vi "Read target.vi"(8 "error in (no error)":errorcluster, 11 "GuideTargetPosition in":refnum<class "GuideTargetPosition.lvclass">) -> (0 "error out":errorcluster, 2 "GWTargetPositionParameters.lvclass":refnum<class "GWTargetPositionParameters.lvclass">, 3 "GuideTargetPosition out":refnum<class "GuideTargetPosition.lvclass">)   [LabVIEW 2014, in "TCSDataDefinitions.lvlib" / "TCSGuiderStatus.lvlib" / "GuideTargetPosition.lvclass"]
uses:
  GuideTargetPosition.lvclass
  GWTargetPositionParameters/GWTargetPositionParameters.lvclass
  GuideTargetPosition.lvclass/GuideTargetPosition.ctl
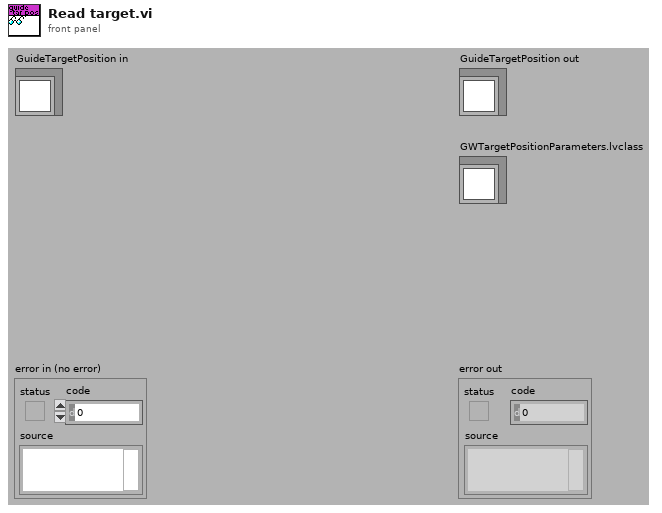
[diagram p1: front panel]
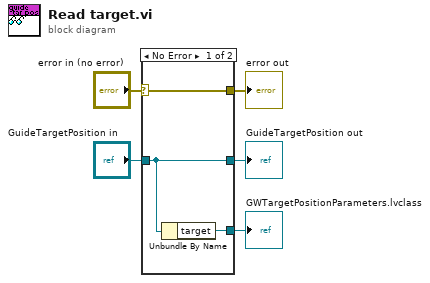
[diagram p0: block diagram]
diagram:
  n1 = case shown="No Error" "error in (no error)" {
    selector: "error in (no error)" -> [w8 w9]
    tunnel: [w8 w9] -> w4
    tunnel: [w7 w10] -> w2
    tunnel: "GuideTargetPosition in" -> [w7 w10]
    tunnel: [w6 _] -> w1
    frame No Error {
      n2 = Unbundle By Name(w7) -> ("target"=w6:refnum<class "GWTargetPositionParameters.lvclass">)
    }
    frame Error {
    }
  }
  "error out" <- w4
  "GuideTargetPosition out" <- w2
  "GWTargetPositionParameters.lvclass" <- w1
